vi "parabola fit2.vi"(8 "radial profile":dbl[](array[numeric])) -> (0 "Y focus":dbl)   [LabVIEW 2011, in "OfflineTracker.lvlib"]
uses:
  OfflineTracker.lvlib
  <vilib>/Analysis/NI_AALPro.lvlib
panel:
  out "Waveform Graph 2":dbl[](graph)
  out "Waveform Graph":dbl[](graph)
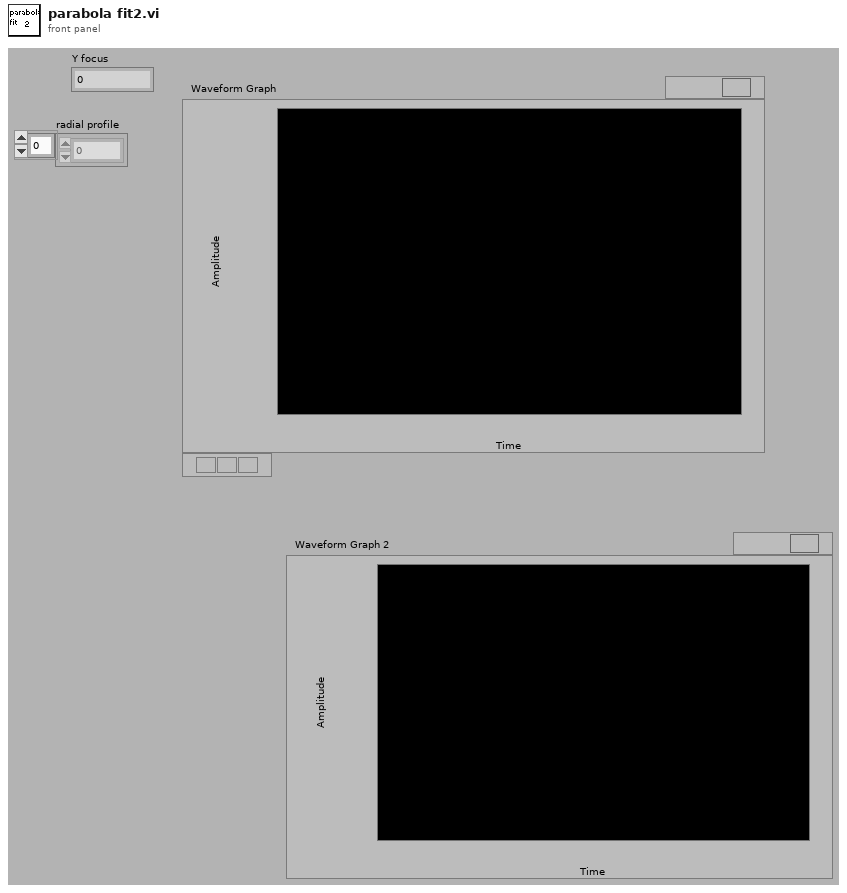
[diagram p1: front panel]
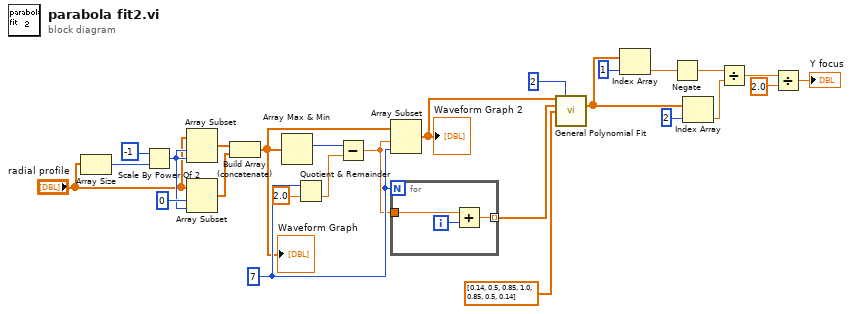
[diagram p0: block diagram]
diagram:
  w15 = 7 ("index")
  n1 = Array Size(array="radial profile") -> (size(s)=w11:i32)
  n2 = Scale By Power Of 2(n=-1, x=w11) -> (x*2^n=w9:i32)
  n3 = Array Subset(array="radial profile", index=w9, length=w9) -> (w8:dbl[])
  n4 = Array Subset(array="radial profile", index=0, length=w9) -> (w7:dbl[])
  n5 = Build Array (concatenate)(w8, w7) -> (w1:dbl[])
  "Waveform Graph" <- w1
  n6 = Array Max & Min(array=w1) -> (max index (indices)=w23:i32)  [unwired: 3 out]
  n7 = Quotient & Remainder(x=w15, y=2.0) -> (floor(x/y)=w16:dbl)  [unwired: 1 out]
  n8 = Subtract(x=w23, y=w16) -> (x-y=w13:dbl)
  n9 = Array Subset(array=w1, index=w13, length=w15) -> (w2:dbl[])
  "Waveform Graph 2" <- w2
  n10 = for {
    N: w15 -> [_]
    tunnel: [w28] -> w3 mode=indexing
    tunnel: w13 -> [w27]
    i -> [w29]
    n11 = Add(x=w27, y=w29) -> (x+y=w28:dbl)
  }
  n12 = call <vilib>:"General Polynomial Fit.vi"("Y"=w2, "polynomial order"=2, "X"=w3, "Weight"=dbl[] [0.14, 0.5, 0.85, 1.0, 0.85, 0.5, 0.14] ("X")) -> ("Polynomial Coefficients"=w4:dbl[])  [unwired: 8 in, 3 out]
  n13 = Index Array(array=w4, index=1 ("Index")) -> (element=w19:dbl)
  n14 = Negate(x=w19) -> (-x=w17:dbl)
  n15 = Index Array(array=w4, index=2 ("Index")) -> (element=w18:dbl)
  n16 = Divide(x=w17, y=w18) -> (x/y=w21:dbl)
  n17 = Divide(x=w21, y=2.0) -> (x/y=→"Y focus":dbl)
